vi "Analog Trigger with Hysteresis (IP).vi"(6 "Reset":bool, 8 "trigger type":enum8{"rising", "falling"}(ring), 9 "hysteresis":i16, 10 "threshold":i16, 11 "signal":i16(slide) scale=0.0..20.0) -> (3 "trigger":bool)   [LabVIEW 2012]
doc: "This VI evaluates the input signal against the trigger parameters to determine if a trigger condition has occured. Before a trigger can (re)occur the signal must go below the threshold minus hysteresis for a rising trigger or above the threshold plus hysteresis for a falling trigger."
panel:
  out "state":bool
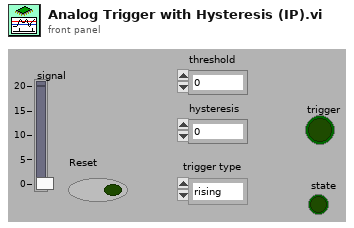
[diagram p1: front panel]
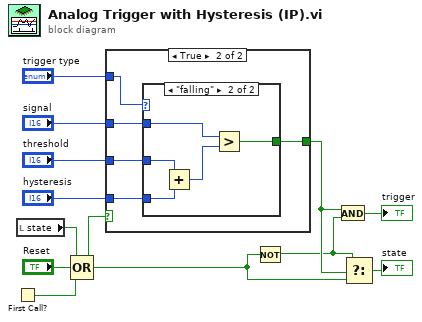
[diagram p0: block diagram]
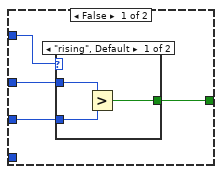
[diagram p2: hidden frame]
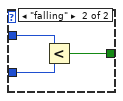
[diagram p3: hidden frame]
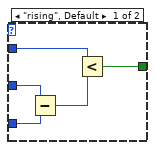
[diagram p4: hidden frame]
diagram:
  n1 = First Call?() -> (First Call?: T/F=w4:bool)
  n2 = local read "state"() -> (w3:bool)
  n3 = Compound Arithmetic op=OR(w3, "Reset", w4) -> (w2:bool)
  n4 = case shown="True" w2 {
    tunnel: "trigger type" -> [w16 w27]
    tunnel: "signal" -> [w15 w26]
    tunnel: "threshold" -> [w14 w25]
    tunnel: "hysteresis" -> [_ w24]
    tunnel: [w13 w23] -> w7
    frame False {
      n5 = case shown="\"rising\", Default" w16 {
        tunnel: w15 -> [w19 w22]
        tunnel: w14 -> [w18 w21]
        tunnel: [w17 w20] -> w13
        frame "rising", Default {
          n6 = Greater?(x=w19, y=w18) -> (0:w17:bool)
        }
        frame "falling" {
          n7 = Less?(x=w22, y=w21) -> (x < y?=w20:bool)
        }
      }
    }
    frame True {
      n8 = case shown="\"falling\"" w27 {
        tunnel: w26 -> [w32 w37]
        tunnel: w25 -> [w30 w34]
        tunnel: w24 -> [w31 w35]
        tunnel: [w28 w33] -> w23
        frame "rising", Default {
          n9 = Subtract(x=w30, y=w31) -> (x-y=w29:i16)
          n10 = Less?(x=w32, y=w29) -> (x < y?=w28:bool)
        }
        frame "falling" {
          n11 = Add(x=w34, y=w35) -> (x+y=w36:i16)
          n12 = Greater?(x=w37, y=w36) -> (0:w33:bool)
        }
      }
    }
  }
  n13 = Not(x=w2) -> (.not. x?=w1:bool)
  n14 = And(x=w7, y=w1) -> (x .and. y?=→"trigger":bool)
  n15 = Select(t=w1, s=w7, f=w2) -> (s? t:f=→"state":bool)
